vi "3d_mesh_test_2.vi"() -> ()   [LabVIEW 2016]
uses:
  <vilib>/picture/3D Picture Control/Object/Create Object (drawable with reference).vi
  <vilib>/picture/3D Picture Control/Object/Add Object (no reference).vi
  <vilib>/picture/3D Picture Control/Helpers/Set Light (reference).vi
  <vilib>/picture/3D Picture Control/NI_3D Picture Control.lvlib
panel:
  in  "Gain":dbl[](array[numeric])=[0.1, 0.1, 0.1]
  in  "Y Coords":dbl[](array[numeric])
  in  "X Coords":dbl[](array[numeric])
  in  "Light State":enum16{"Inherit Value", "Off", "On"}(ring)=enum."On"
  in  "Stop":bool
  out "3D Picture":refnum<vi>(3d-picture)
  in  "Light Direction":cluster{"X":sgl, "Y":sgl, "Z":sgl}={"X"=0.0, "Y"=0.0, "Z"=-1.0}
  in  "Light Colour":u32(colorbox)=16711680
  in  "Radius":sgl=0.01
  in  "Length":sgl=2.0
  in  "Character Size":sgl=0.5
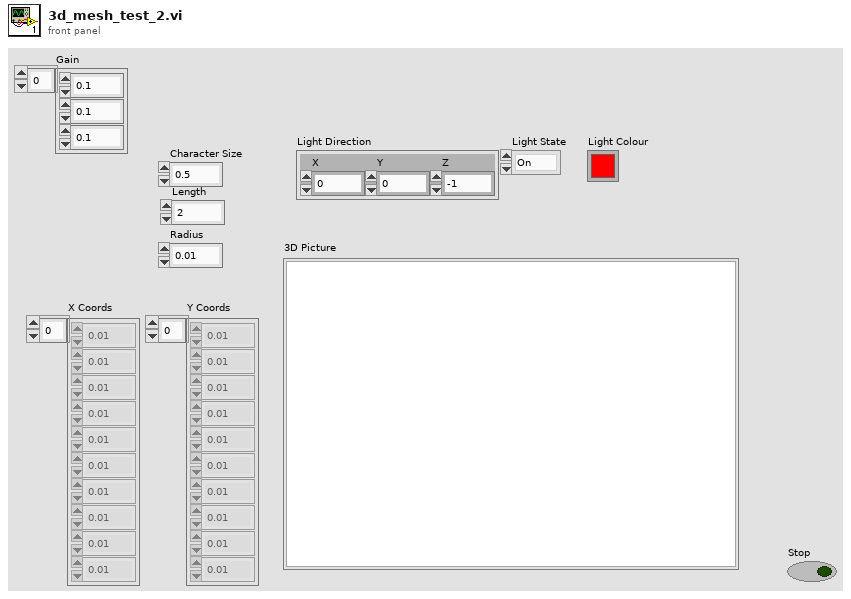
[diagram p1: front panel]
types:
  T1 = typedef "3D_Plot_Data.ctl" = cluster{"Size":i32[], "Gain":dbl[], "X Baseline":dbl[][], "Y Baseline":dbl[][], "Z Baseline":dbl[][], "SceneMesh out":refnum<vi>}
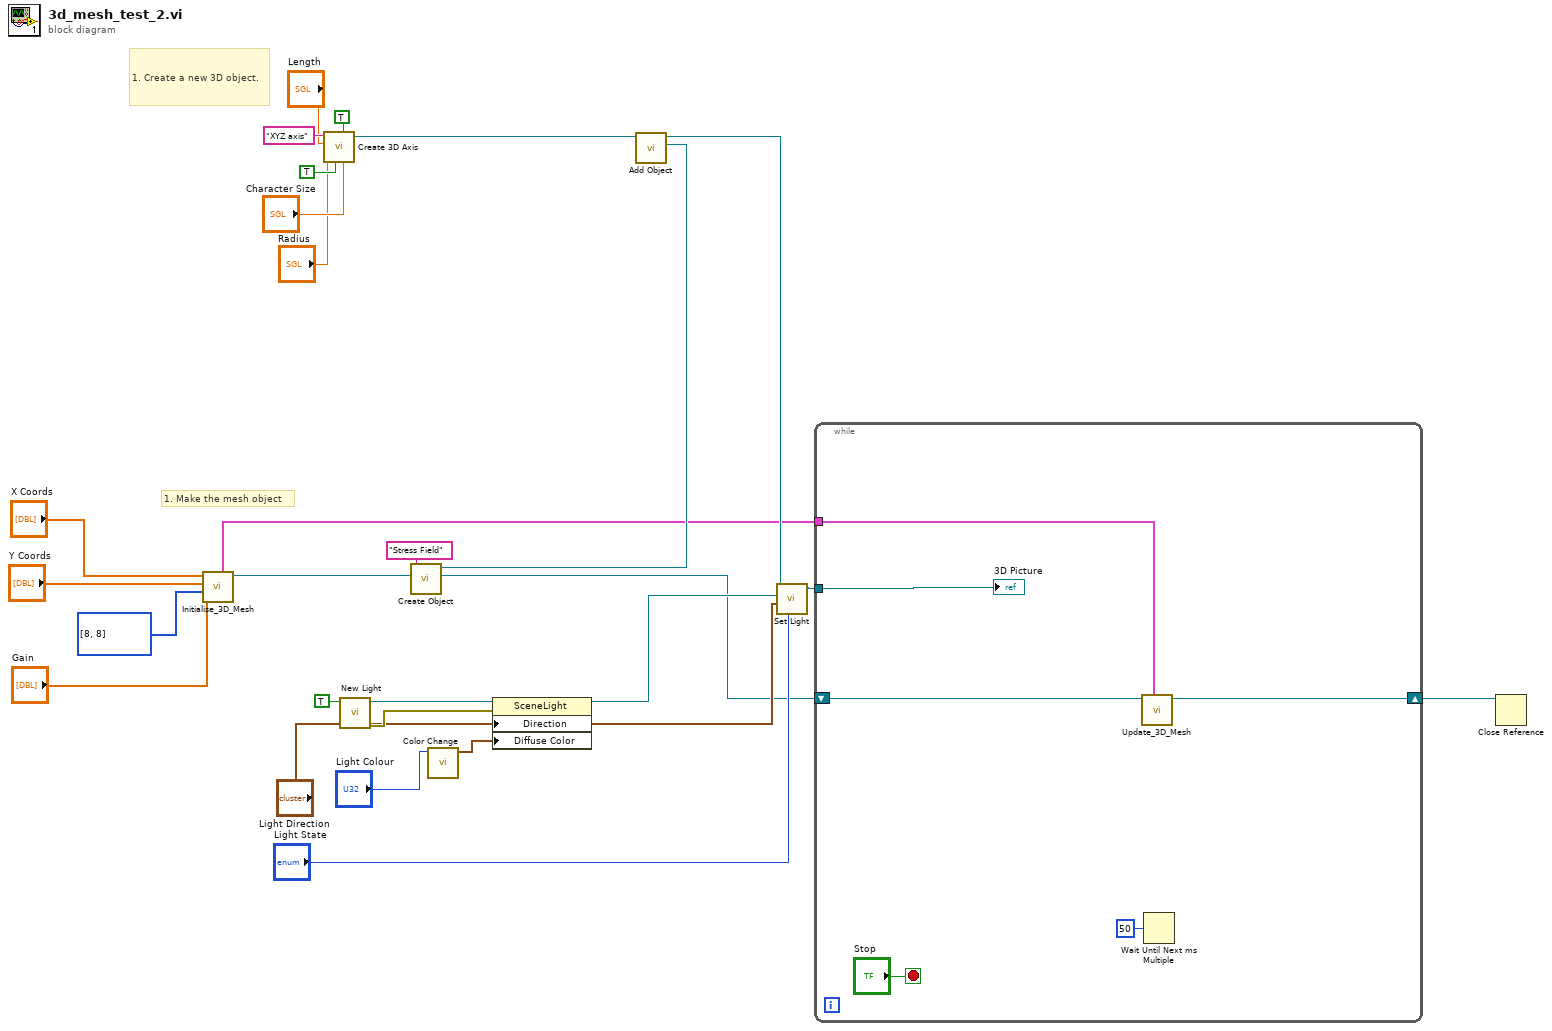
[diagram p0: block diagram]
diagram:
  # "1. Make the mesh object"
  # "1. Create a new 3D object."
  n1 = call "Initialise_3D_Mesh.vi"("Gain"="Gain", "Size"=i32[] [8, 8], "Y Coords"="Y Coords", "X Coords"="X Coords") -> ("SceneMesh out"=w9:refnum<vi>, "3D Plot Data"=w1:T1)  [unwired: 6 in]
  n2 = call <vilib>:"Create 3D Axis.vi"("Character Size"="Character Size", "Half plane?"=TRUE, "Axis label?"=TRUE, "Radius"="Radius", "Length"="Length", "Name"="XYZ axis") -> ("New Object Refnum"=w21:refnum<vi>)  [unwired: 4 in, 1 out]
  n3 = call <vilib>:"New Light.vi"("At Infinity"=TRUE) -> ("error out"=w24:errorcluster, "New Light Refnum"=w27:refnum<vi>)  [unwired: 2 in, 7 out]
  n4 = call-poly <vilib>:"Create Object.vi"("Geometry or text"=w9, "Name"="Stress Field") -> ("Drawable refnum"=w6:refnum<vi>, "Scene:New Object"=w7:refnum<vi>)  [unwired: 7 in, 1 out]
  n5 = call <vilib>:"Color Change.vi"("Color"="Light Colour") -> ("RGBA"=w23:cluster{"R":sgl, "G":sgl, "B":sgl, "A":sgl})  [unwired: 10 in]
  n6 = property class="SceneLight"(reference=w27, error in=w24, "Direction"="Light Direction", "Diffuse Color"=w23) -> (reference out=w10:refnum<vi>)  [unwired: 1 out]
  n7 = call-poly <vilib>:"Add Object.vi"("New Object In"=w7, "Scene Object In"=w21) -> ("Scene Object Out"=w12:refnum<vi>)  [unwired: 8 in, 1 out]
  n8 = call-poly <vilib>:"Set Light.vi"("Light State"="Light State", "Position"="Light Direction", "Light Refnum In"=w10, "Scene Object In"=w12) -> ("Scene Object Out"=w11:refnum<vi>)  [unwired: 5 in, 2 out]
  n9 = while {
    tunnel: w11 -> [w33]
    shift-right: [w29] -> w8
    shift-left: w6 -> [w30]
    tunnel: w1 -> [w28]
    stop <- "Stop" stop-if-true
    n10 = call "Update_3D_Mesh.vi"("3D Plot Data"=w28, "SceneDrawable in"=w30) -> ("SceneDrawable out"=w29:refnum<vi>)  [unwired: 9 in]
    n11 = Wait Until Next ms Multiple(millisecond multiple=u32 50) -> ()  [unwired: 1 out]
    "3D Picture" <- w33
  }
  n12 = Close Reference(reference=w8) -> ()  [unwired: 1 in, 1 out]
